vi "EvaluacionTabla.vi"(8 "error in (no error)":errorcluster, 10 "Cluster":cluster{"Tabla":string, "Posicion":T1}, 11 "Prueba33 in":refnum<class "Prueba33.lvclass">) -> (0 "error out":errorcluster, 3 "Prueba33 out":refnum<class "Prueba33.lvclass">)   [LabVIEW 2019, in "Prueba33.lvclass"]
uses:
  Prueba33.lvclass
  <vilib>/Utility/miscctls.llb/LVRowAndColumnTypeDef.ctl
  Prueba33.lvclass/Prueba33.ctl
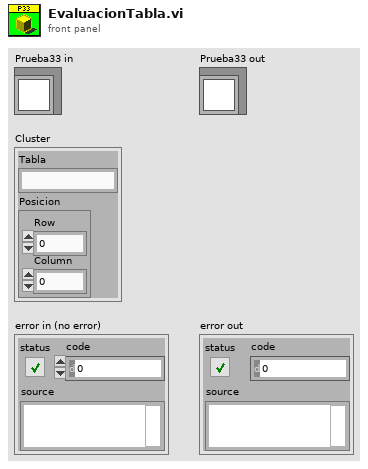
[diagram p1: front panel]
types:
  T1 = typedef "LVRowAndColumnTypeDef.ctl" = cluster{"Row":i32, "Column":i32}
  T2 = cluster{"ControlName":string, "ControlReference":refnum<vi>}[]
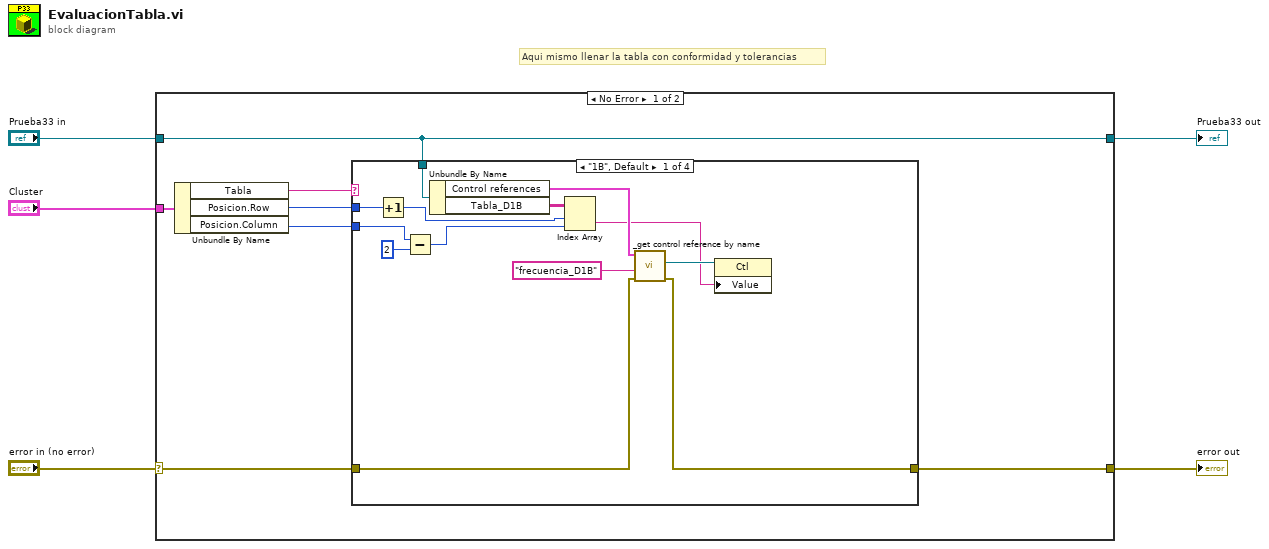
[diagram p0: block diagram]
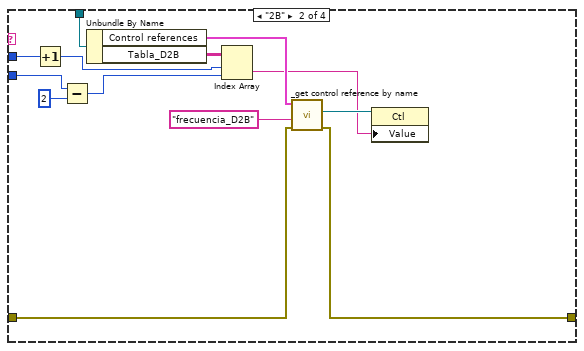
[diagram p2: hidden frame]
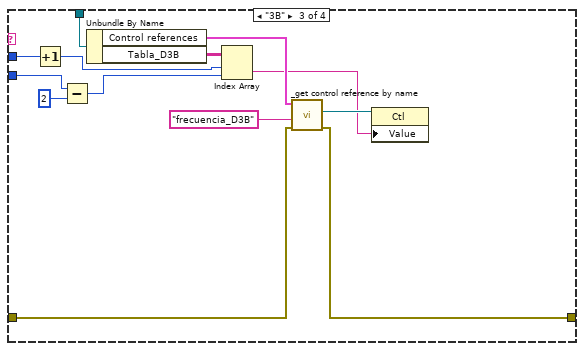
[diagram p3: hidden frame]
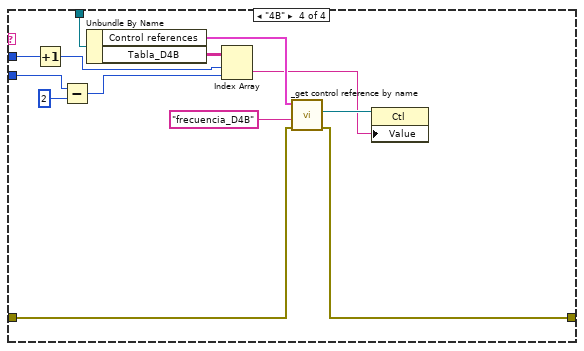
[diagram p4: hidden frame]
diagram:
  # "Aqui mismo llenar la tabla con conformidad y tolerancias"
  n1 = case shown="No Error" "error in (no error)" {
    selector: "error in (no error)" -> [w7 w65]
    tunnel: [w6 w65] -> w2
    tunnel: [w11 w66] -> w4
    tunnel: "Prueba33 in" -> [w11 w66]
    tunnel: "Cluster" -> [w12 _]
    frame No Error {
      n2 = Unbundle By Name(w12) -> ("Tabla"=w10:string, "Posicion.Row"=w9:i32, "Posicion.Column"=w8:i32)
      n3 = case shown="\"1B\", Default" w10 {
        tunnel: w11 -> [w25 w38 w51 w64]
        tunnel: w9 -> [w23 w36 w49 w62]
        tunnel: w8 -> [w14 w27 w40 w53]
        tunnel: w7 -> [w20 w33 w46 w59]
        tunnel: [w19 w32 w45 w58] -> w6
        frame "1B", Default {
          n4 = Increment(x=w23) -> (x+1=w16:i32)
          n5 = Subtract(x=w14, y=2) -> (x-y=w15:i32)
          n6 = Unbundle By Name(w25) -> ("Control references"=w22:T2, "Tabla_D1B"=w24:string[][])
          n7 = Index Array(array=w24, index (row)=w16, index (col)=w15) -> (element=w17:string)
          n8 = call "_get control reference by name.vi"("error in (no error)"=w20, "Control name"="frecuencia_D1B", "Control references"=w22) -> ("error out"=w19:errorcluster, "Ctl Refnum"=w18:refnum<vi>)  [unwired: 3 in]
          n9 = property class="Ctl"(reference=w18, "Value"=w17) -> ()  [unwired: 1 in, 2 out]
        }
        frame "2B" {
          n10 = Increment(x=w36) -> (x+1=w29:i32)
          n11 = Subtract(x=w27, y=2) -> (x-y=w28:i32)
          n12 = Unbundle By Name(w38) -> ("Control references"=w35:T2, "Tabla_D2B"=w37:string[][])
          n13 = Index Array(array=w37, index (row)=w29, index (col)=w28) -> (element=w30:string)
          n14 = call "_get control reference by name.vi"("error in (no error)"=w33, "Control name"="frecuencia_D2B", "Control references"=w35) -> ("error out"=w32:errorcluster, "Ctl Refnum"=w31:refnum<vi>)  [unwired: 3 in]
          n15 = property class="Ctl"(reference=w31, "Value"=w30) -> ()  [unwired: 1 in, 2 out]
        }
        frame "3B" {
          n16 = Increment(x=w49) -> (x+1=w42:i32)
          n17 = Subtract(x=w40, y=2) -> (x-y=w41:i32)
          n18 = Unbundle By Name(w51) -> ("Control references"=w48:T2, "Tabla_D3B"=w50:string[][])
          n19 = Index Array(array=w50, index (row)=w42, index (col)=w41) -> (element=w43:string)
          n20 = call "_get control reference by name.vi"("error in (no error)"=w46, "Control name"="frecuencia_D3B", "Control references"=w48) -> ("error out"=w45:errorcluster, "Ctl Refnum"=w44:refnum<vi>)  [unwired: 3 in]
          n21 = property class="Ctl"(reference=w44, "Value"=w43) -> ()  [unwired: 1 in, 2 out]
        }
        frame "4B" {
          n22 = Increment(x=w62) -> (x+1=w55:i32)
          n23 = Subtract(x=w53, y=2) -> (x-y=w54:i32)
          n24 = Unbundle By Name(w64) -> ("Control references"=w61:T2, "Tabla_D4B"=w63:string[][])
          n25 = Index Array(array=w63, index (row)=w55, index (col)=w54) -> (element=w56:string)
          n26 = call "_get control reference by name.vi"("error in (no error)"=w59, "Control name"="frecuencia_D4B", "Control references"=w61) -> ("error out"=w58:errorcluster, "Ctl Refnum"=w57:refnum<vi>)  [unwired: 3 in]
          n27 = property class="Ctl"(reference=w57, "Value"=w56) -> ()  [unwired: 1 in, 2 out]
        }
      }
    }
    frame Error {
    }
  }
  "Prueba33 out" <- w4
  "error out" <- w2
